vi "MockGyro.vi"(11 "MockGyroData":T1={"BufferUpdateFIFO"="MockGyroBufferUpdate", "MockGyroCommandInput"="ModbusSubnetEGyroRxDataFIFO", "MockGyroDataOutput"="ModbusSubnetEGyroTxDataFIFO", "MockGyroDataRate"="MockGyroDataRateRegister", "MockGyroXValue"="MockGyroXValueRegister", "MockGyroYValue"="MockGyroYValueRegister", "MockGyroZValue"="MockGyroZValueRegister", "MockGyroStatus"="MockGyroStatusRegister", "MockGyroTemperature"="MockGyroTemperatureRegister", "CRCDataFIFO"="MockGyroCRCDataFIFO", "CRCCalculateFIFO"="MockGyroCRCCalculateFIFO", "CRCFIFO"="MockGyroCRCFIFO", "MockGyroCommandReplyFIFO"="MockGyroCommandReplyFIFO", "MockGyroReplyReadyFIFO"="MockGyroReplyReadyFIFO", "MockGyroModeFIFO"="MockGyroModeFIFO"}) -> ()   [LabVIEW 2016, in "FPGAMockGyro.lvlib"]
uses:
  FPGAMockGyro.lvlib
  Common_FPGA_Modbus/FPGAModbus.lvlib
  Common_FPGA_Modbus/DataTypes/ModbusCRC32Settings.ctl
  DataTypes/MockGyroData.ctl
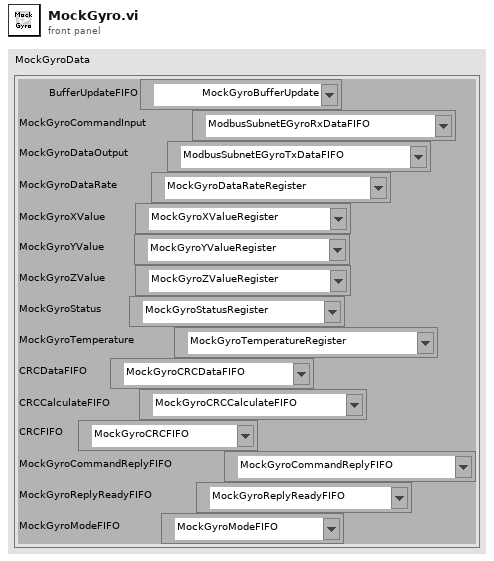
[diagram p1: front panel]
types:
  T1 = typedef "FPGAMockGyro.lvlib/MockGyroData.ctl" = cluster{"BufferUpdateFIFO":refnum<k21>, "MockGyroCommandInput":refnum<k21>, "MockGyroDataOutput":refnum<k21>, "MockGyroDataRate":refnum<k21>, "MockGyroXValue":refnum<k21>, "MockGyroYValue":refnum<k21>, "MockGyroZValue":refnum<k21>, "MockGyroStatus":refnum<k21>, "MockGyroTemperature":refnum<k21>, "CRCDataFIFO":refnum<k21>, "CRCCalculateFIFO":refnum<k21>, "CRCFIFO":refnum<k21>, "MockGyroCommandReplyFIFO":refnum<k21>, "MockGyroReplyReadyFIFO":refnum<k21>, "MockGyroModeFIFO":refnum<k21>}
  T2 = typedef "FPGAModbus.lvlib/ModbusCRC32Settings.ctl" = cluster{"DataFIFO":refnum<k21>, "CalculateFIFO":refnum<k21>, "OutputFIFO":refnum<k21>}
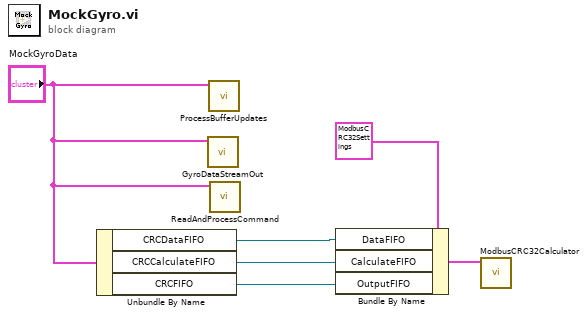
[diagram p0: block diagram]
diagram:
  n1 = Unbundle By Name("MockGyroData") -> ("CRCDataFIFO"=w2:refnum<k21>, "CRCCalculateFIFO"=w6:refnum<k21>, "CRCFIFO"=w1:refnum<k21>)
  n2 = call "GyroDataStreamOut.vi"("MockGyroData"="MockGyroData") -> ()  [unwired: 11 in]
  n3 = call "ProcessBufferUpdates.vi"("MockGyroData"="MockGyroData") -> ()  [unwired: 11 in]
  n4 = call "ReadAndProcessCommand.vi"("MockGyroData In"="MockGyroData") -> ()  [unwired: 11 in]
  n5 = Bundle By Name(cluster=T2 {"DataFIFO"="MockGyroCRCDataFIFO", "CalculateFIFO"="MockGyroCRCCalculateFIFO", "OutputFIFO"="MockGyroCRCFIFO"} ("ModbusCRC32Settings"), "DataFIFO"=w2, "CalculateFIFO"=w6, "OutputFIFO"=w1) -> (w5:T2)
  n6 = call "ModbusCRC32Calculator.vi"("ModbusCRC32Settings"=w5) -> ()  [unwired: 11 in]
